vi "ui_launcher.vi"   [LabVIEW 2015]
uses:
  front_panel_class/front_panel.lvclass
  <vilib>/ActorFramework/Actor/Actor.lvclass
panel:
  # "Start to launch the PCFS GUI"
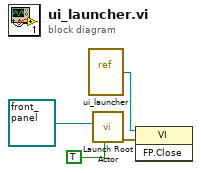
[diagram p0: block diagram]
diagram:
  n1 = vi-ref "ui_launcher.vi"() -> (w2:refnum<vi>)
  n2 = call <vilib>:"Launch Root Actor.vi"("Open Actor Core front panel? (F)"=TRUE, "Actor"=refnum<class "front_panel.lvclass"> refnum ("front_panel.lvclass")) -> ("error out"=w3:errorcluster)  [unwired: 8 in, 1 out]
  n3 = invoke class="VI" method="FP.Close"(reference=w2, error in=w3) -> ()  [unwired: 1 in, 3 out]
